vi "LVIS_Log.vi"(8 "Error In":errorcluster) -> (0 "Error Out":errorcluster)   [LabVIEW 2015]
doc: "Displays the event data that would potentially be sent to the Data Commander"
uses:
  Globals/LVIS_DcGlobals.vi
panel:
  out "Event Log":string[][](table)
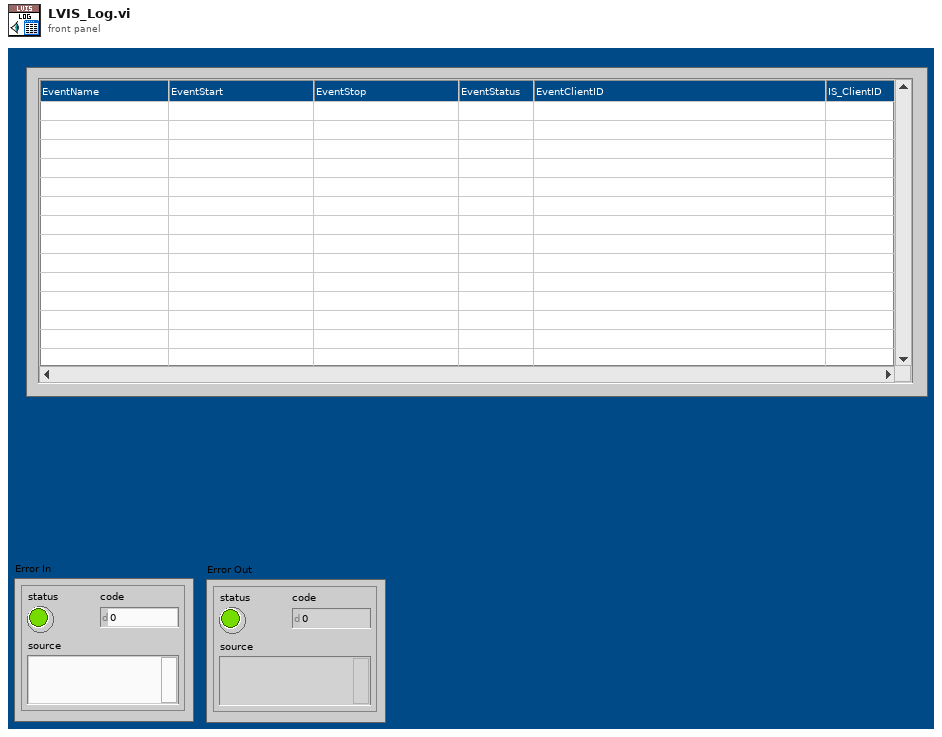
[diagram p1: front panel]
types:
  T1 = enum32{"Invalid", "Standard", "Closed", "Hidden", "Minimized", "Maximized"}
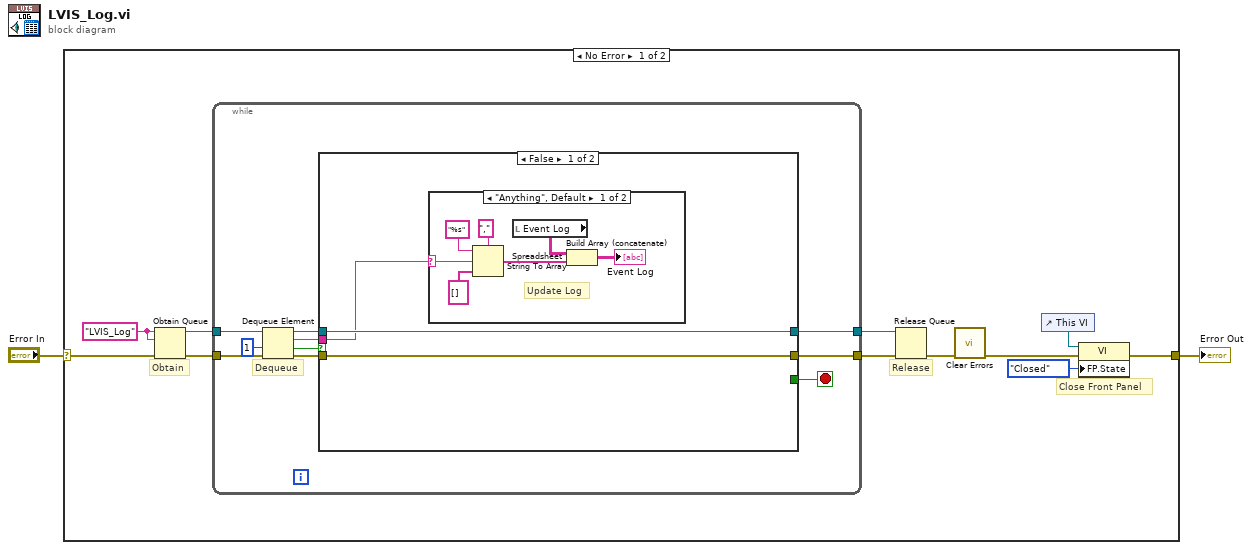
[diagram p0: block diagram]
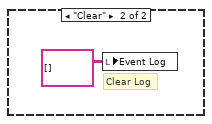
[diagram p2: hidden frame]
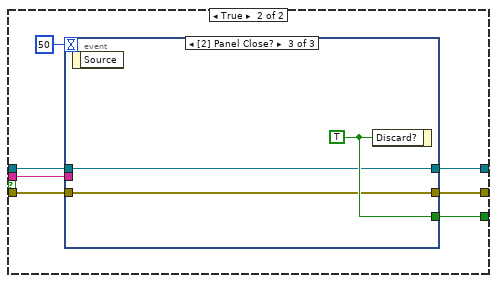
[diagram p3: hidden frame]
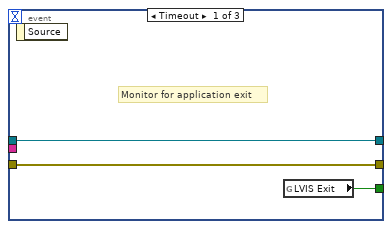
[diagram p4: hidden frame]
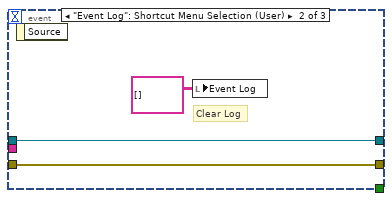
[diagram p5: hidden frame]
diagram:
  n1 = case shown="No Error" "Error In" {
    selector: "Error In" -> [w13 w51]
    tunnel: [w5 w51] -> w1
    frame No Error {
      w12 = "LVIS_Log" ("name (unnamed)")
      # "Close Front Panel"
      # "Release"
      # "Obtain"
      n2 = Obtain Queue(name (unnamed)=w12, element data type=w12, error in (no error)=w13) -> (queue out=w10:refnum<queue>, error out=w11:errorcluster)  [unwired: 2 in, 1 out]
      n3 = while {
        tunnel: w11 -> [w21]
        tunnel: [w23] -> w9
        tunnel: w10 -> [w19]
        tunnel: [w14] -> w8
        stop <- w22 stop-if-true
        # "Dequeue"
        n4 = Dequeue Element(queue=w19, timeout in ms (-1)=1, error in (no error)=w21) -> (queue out=w17:refnum<queue>, element=w16:string, timed out?=w15:bool, error out=w20:errorcluster)
        n5 = case shown="False" w15 {
          tunnel: [w26 w41] -> w23
          tunnel: [_ w40] -> w22
          tunnel: w20 -> [w26 w38]
          tunnel: w17 -> [w25 w37]
          tunnel: w16 -> [w24 w36]
          tunnel: [w25 w35] -> w14
          frame False {
            n6 = case shown="\"Anything\", Default" w24 {
              selector: w24 -> [w27 _]
              frame "Anything", Default {
                # "Update Log"
                n7 = Spreadsheet String To Array(delimiter (Tab)=",", format string="%s", spreadsheet string=w27, array type (2D Dbl)=string[] []) -> (array=w31:string[])
                n8 = local read "Event Log"() -> (w32:string[][])
                n9 = Build Array (concatenate)(w32, w31) -> (→"Event Log":string[][])
              }
              frame "Clear" {
                # "Clear Log"
                n10 = local write "Event Log"(string[][] [] ("Event Log")) -> ()
              }
            }
          }
          frame True {
            n11 = event shown="[2] Panel Close?" {
              selector: _ -> [_ _ _]
              dyn-events: _ -> [_ _ _]
              timeout: 50 -> [_ _ _]
              tunnel: w38 -> [w43 w47 w48]
              tunnel: [w43 w47 w48] -> w41
              tunnel: [w44 _ w50] -> w40
              tunnel: w37 -> [w42 w45 w49]
              tunnel: w36 -> [_ _ _]
              tunnel: [w42 w45 w49] -> w35
              event Timeout {
                # "Monitor for application exit"
                n12 = event-data() -> ()  [unwired: 1 in, 1 out]
                n13 = global read "LVIS_DcGlobals.vi" "LVIS Exit"() -> (w44:bool)
              }
              event "Event Log": Shortcut Menu Selection (User) {
                # "Clear Log"
                n14 = event-data() -> ()  [unwired: 1 in, 1 out]
                n15 = local write "Event Log"(string[][] [] ("Event Log")) -> ()
              }
              event Panel Close? {
                w50 = TRUE ("Discard?")
                n16 = event-data() -> ()  [unwired: 1 in, 1 out]
                n17 = event-data("Discard?"=w50) -> ()  [unwired: 1 in, 1 out]
              }
            }
          }
        }
      }
      n18 = Release Queue(queue=w8, error in (no error)=w9) -> (error out=w4:errorcluster)  [unwired: 1 in, 2 out]
      n19 = call <vilib>:"Clear Errors.vi"("error in (no error)"=w4) -> ("error out"=w3:errorcluster)  [unwired: 5 in, 1 out]
      n20 = control-ref of="This VI"() -> (w7:refnum<vi>)
      n21 = property class="VI"(reference=w7, error in=w3, "FP.State"=T1."Closed" ("Front Panel Window:State")) -> (error out=w5:errorcluster)  [unwired: 1 out]
    }
    frame Error {
    }
  }
  "Error Out" <- w1
